vi "Check for Node Existence.vi"(8 "error in (no error)":errorcluster, 10 "XPath Expression":string, 11 "Node to Search":refnum<k20>) -> (0 "error out":errorcluster, 2 "Exists?":bool, 3 "Node to Search out":refnum<k20>)   [LabVIEW 2013]
uses:
  <vilib>/xml/Close Reference(Node).vi
  <vilib>/xml/NI_XML.lvlib
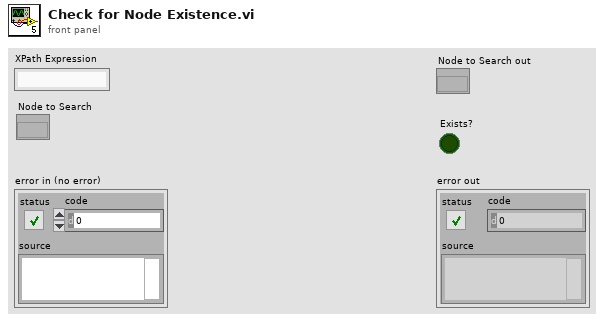
[diagram p1: front panel]
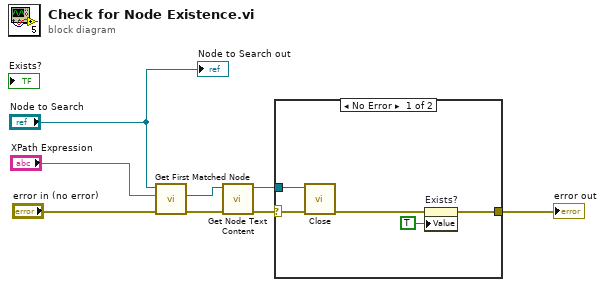
[diagram p0: block diagram]
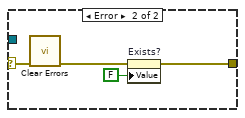
[diagram p2: hidden frame]
diagram:
  n1 = call <vilib>:"Get First Matched Node.vi"("error in (no error)"="error in (no error)", "XPath expression"="XPath Expression", "node in"="Node to Search") -> ("error out"=w7:errorcluster, "node result"=w8:refnum<k20>)  [unwired: 6 in, 1 out]
  n2 = call <vilib>:"Get Node Text Content.vi"("error in (no error)"=w7, "node in"=w8) -> ("error out"=w4:errorcluster, "node out"=w3:refnum<k20>)  [unwired: 7 in, 1 out]
  n3 = case shown="No Error" w4 {
    selector: w4 -> [w11 w17]
    tunnel: [w13 w15] -> w2
    tunnel: w3 -> [w10 _]
    frame No Error {
      n4 = call-poly <vilib>:"Close.vi"("error in (no error)"=w11, "node"=w10) -> ("error out"=w9:errorcluster)  [unwired: 7 in]
      n5 = property on="Exists?" class="Bool (strict)"(error in=w9, "Value"=TRUE ("Exists?")) -> (error out=w13:errorcluster)  [unwired: 1 in, 1 out]
    }
    frame Error {
      n6 = call <vilib>:"Clear Errors.vi"("error in (no error)"=w17) -> ("error out"=w16:errorcluster)  [unwired: 6 in]
      n7 = property on="Exists?" class="Bool (strict)"(error in=w16, "Value"=FALSE ("Exists?")) -> (error out=w15:errorcluster)  [unwired: 1 in, 1 out]
    }
  }
  "error out" <- w2
  "Node to Search out" <- "Node to Search"
